vi "Print PDF.vi"(6 "Timeout ms":i32=10000, 8 "error in (no error)":errorcluster, 9 "PDF File Path":path, 10 "printSettings":refnum<k24>, 11 "WebView2 Control in":refnum<class "WebView2 QControl.lvclass">) -> (0 "error out":errorcluster, 2 "Timeout":bool, 3 "WebView2 Control out":refnum<class "WebView2 QControl.lvclass">)   [LabVIEW 2020, in "WebView2 QControl.lvlib" / "WebView2 QControl.lvclass"]
uses:
  WebView2 QControl.lvclass
  C:/Users/Simon/Documents/GitHub/LV-WebView2/Source/Libs/Microsoft.Web.WebView2.Core.dll
  Libs/Microsoft.Web.WebView2.Core.dll
  WebView2 QControl.lvclass/WebView2 QControl.ctl
  Webview2 Lib/WebView2 Control Object/WebView2 Control.lvclass
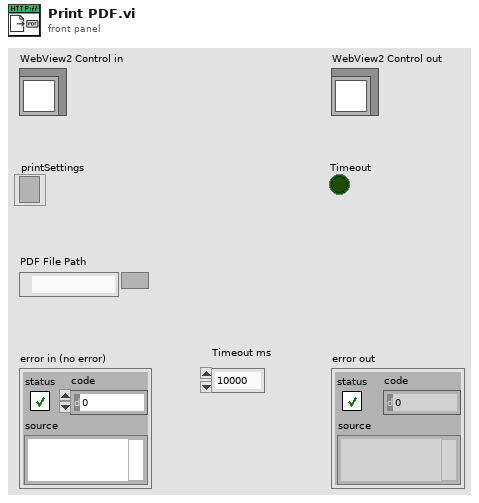
[diagram p1: front panel]
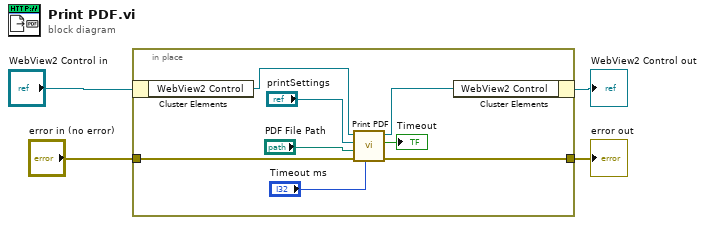
[diagram p0: block diagram]
diagram:
  n1 = in-place {
    in-place-border: "error in (no error)" -> [w12]
    in-place-border: [w11] -> w1
    n2 = in-place-cluster #1("WebView2 Control in") -> ("WebView2 Control"=w10:refnum<class "WebView2 Control.lvclass">)
    n3 = call "Print PDF.vi"("Timeout ms"="Timeout ms", "error in (no error)"=w12, "PDF File Path"="PDF File Path", "printSettings"="printSettings", "WebView2 Control in"=w10) -> ("error out"=w11:errorcluster, "Timeout"=→"Timeout":bool, "WebView2 Control out"=w9:refnum<class "WebView2 Control.lvclass">)  [unwired: 4 in]
    n4 = in-place-cluster #1("WebView2 Control"=w9) -> (→"WebView2 Control out":refnum<class "WebView2 QControl.lvclass">)
  }
  "error out" <- w1
